vi "CAN_Receive.vi"(8 "错误输入（无错误）":errorcluster, 9 "WaitTime":i32, 10 "Length":u32, 11 "General_Input":T2) -> (0 "错误输出":errorcluster, 2 "VCI_CAN_OBJ_R":T3 {"Reserved 2" format="%x"; "Reserved 1" format="%x"; "Reserved 0" format="%x"; "Data 7" format="%x"; "Data 6" format="%x"; "Data 5" format="%x"; "Data 4" format="%x"; "Data 3" format="%x"; "Data 2" format="%x"; "Data 1" format="%x"; "Data 0" format="%x"; "DataLen" format="%x"; "ExternFlag" format="%x"; "RemoteFlag" format="%x"; "SendType" format="%x"; "TimeFlag" format="%x"; "TimeStamp" format="%x"; "ID" format="%x"}, 3 "General_Output":T1)   [LabVIEW 2012]
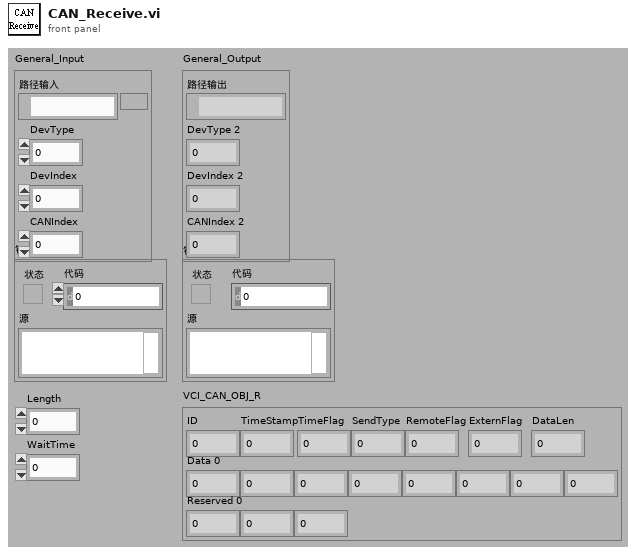
[diagram p1: front panel]
types:
  T1 = cluster{"路径输出":path, "DevType 2":u32, "DevIndex 2":u32, "CANIndex 2":u32}
  T2 = cluster{"路径输入":path, "DevType":u32, "DevIndex":u32, "CANIndex":u32}
  T3 = cluster{"ID":u32, "TimeStamp":u32, "TimeFlag":u8, "SendType":u8, "RemoteFlag":u8, "ExternFlag":u8, "DataLen":u8, "Data 0":u8, "Data 1":u8, "Data 2":u8, "Data 3":u8, "Data 4":u8, "Data 5":u8, "Data 6":u8, "Data 7":u8, "Reserved 0":u8, "Reserved 1":u8, "Reserved 2":u8}
  T4 = cluster{"path out":path, "DevType":u32, "DevIndex":u32, "CANIndex":u32}
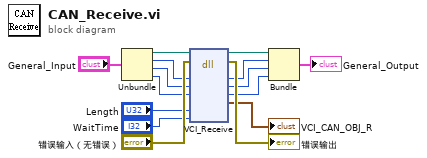
[diagram p0: block diagram]
diagram:
  n1 = Unbundle("General_Input") -> ("路径输入"=w9:path, "DevType"=w6:u32, "DevIndex"=w7:u32, "CANIndex"=w8:u32)
  n2 = dll-call lib="?" fn="VCI_Receive"(path in=w9, error in="错误输入（无错误）", "DevType"=w6, "DevIndex"=w7, "CANIndex"=w8, "Length"="Length", "WaitTime"="WaitTime") -> (path out=w5:path, error out=→"错误输出":errorcluster, "DevType"=w2:u32, "DevIndex"=w3:u32, "CANIndex"=w4:u32, "VCI_CAN_OBJ_R"=→"VCI_CAN_OBJ_R":T3)  [unwired: 5 in]
  n3 = Bundle("path out"=w5, "DevType"=w2, "DevIndex"=w3, "CANIndex"=w4) -> (→"General_Output":T4)  [unwired: 1 in]
